vi "FV_motor_status.vi"(7 "do_reset":bool, 8 "error in":errorcluster, 11 "VISA":refnum<visa-resource-name>) -> (0 "error out":errorcluster, 1 "motor_alarm":i32, 2 "motor_status":i32, 3 "VISA out":refnum<visa-resource-name>, 4 "status":bool, 5 "is_on":bool)   [LabVIEW 2019]
panel:
  out "return_AL":string
  out "return_SC":string
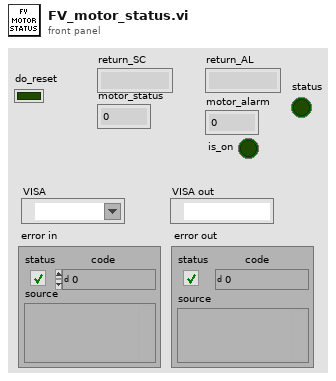
[diagram p1: front panel]
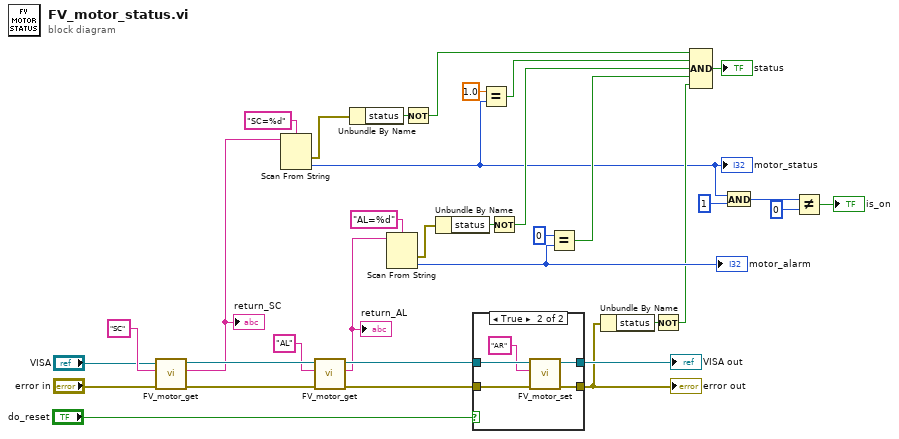
[diagram p0: block diagram]
diagram:
  n1 = call "FV_motor_get.vi"("error in"="error in", "command"="SC", "VISA in"="VISA") -> ("error out"=w31:errorcluster, "return"=w24:string, "VISA out"=w30:refnum<visa-resource-name>)  [unwired: 5 in, 1 out]
  "return_SC" <- w24
  n2 = Scan From String(format string="SC=%d", input string=w24) -> (error out=w20:errorcluster, output 1=w1:i32)  [unwired: 3 in, 2 out]
  "motor_status" <- w1
  n3 = call "FV_motor_get.vi"("error in"=w31, "command"="AL", "VISA in"=w30) -> ("error out"=w26:errorcluster, "return"=w22:string, "VISA out"=w27:refnum<visa-resource-name>)  [unwired: 5 in, 1 out]
  "return_AL" <- w22
  n4 = Unbundle By Name(w20) -> ("status"=w17:bool)
  n5 = Scan From String(format string="AL=%d", input string=w22) -> (error out=w19:errorcluster, output 1=w11:i32)  [unwired: 3 in, 2 out]
  "motor_alarm" <- w11
  n6 = Not(x=w17) -> (.not. x?=w16:bool)
  n7 = Unbundle By Name(w19) -> ("status"=w15:bool)
  n8 = case shown="True" "do_reset" {
    tunnel: w27 -> [w36 w41]
    tunnel: w26 -> [w35 w40]
    tunnel: [w35 w39] -> w8
    tunnel: [w36 w38] -> w25
    frame False {
    }
    frame True {
      n9 = call "FV_motor_set.vi"("error in"=w40, "command"="AR", "VISA in"=w41) -> ("error out"=w39:errorcluster, "VISA out"=w38:refnum<visa-resource-name>)  [unwired: 7 in]
    }
  }
  "error out" <- w8
  "VISA out" <- w25
  n10 = Equal?(x=1.0, y=w1) -> (x = y?=w12:bool)
  n11 = Not(x=w15) -> (.not. x?=w13:bool)
  n12 = Equal?(x=0, y=w11) -> (x = y?=w9:bool)
  n13 = Unbundle By Name(w8) -> ("status"=w7:bool)
  n14 = Not(x=w7) -> (.not. x?=w6:bool)
  n15 = Compound Arithmetic op=AND(w16, w12, w13, w9, w6) -> (→"status":bool)
  n16 = And(x=w1, y=1) -> (x .and. y?=w3:i32)
  n17 = Not Equal?(x=w3, y=0) -> (x != y?=→"is_on":bool)
